vi "Dependency Add Source Path.vi"(7 "Source Path (relative)":string, 8 "error in (no error)":errorcluster, 10 "Dependency ref in":refnum<k20>, 11 "XML File ref in":refnum<k20>) -> (0 "error out":errorcluster, 2 "Dependency ref out":refnum<k20>, 3 "XML File ref out":refnum<k20>)   [LabVIEW 2020, in "LVLIBP CD XML Updater.lvlib" / "Project XML Editor.lvclass"]
uses:
  Project XML Editor.lvclass
  <vilib>/xml/Close Reference(Node).vi
  <resource>/objmgr/DOMUserDefRef.rc
  <vilib>/xml/NI_XML.lvlib
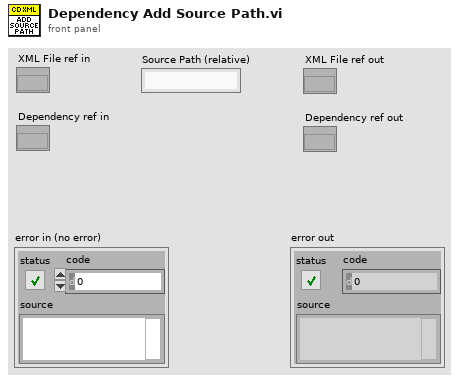
[diagram p1: front panel]
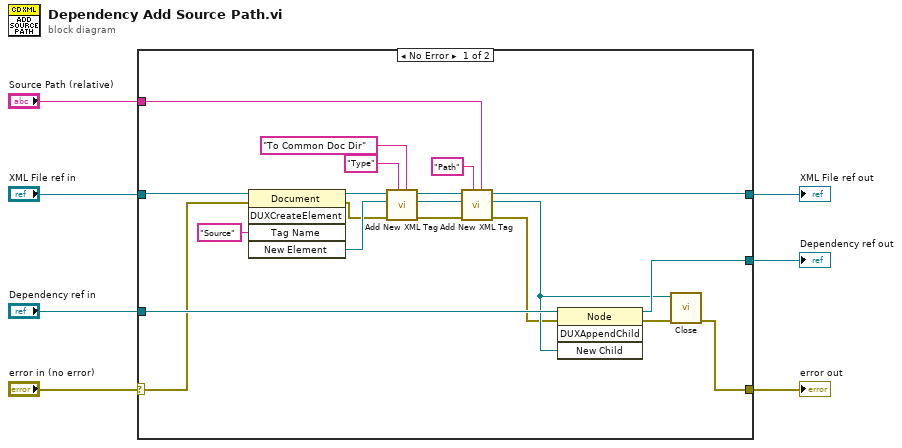
[diagram p0: block diagram]
diagram:
  n1 = case shown="No Error" "error in (no error)" {
    selector: "error in (no error)" -> [w13 w28]
    tunnel: "Source Path (relative)" -> [w19 _]
    tunnel: "XML File ref in" -> [w20 w29]
    tunnel: "Dependency ref in" -> [w18 w30]
    tunnel: [w17 w30] -> w4
    tunnel: [w16 w29] -> w3
    tunnel: [w9 w28] -> w2
    frame No Error {
      n2 = invoke class="Document" method="DUXCreateElement"(reference=w20, error in=w13, "Tag Name"="Source") -> (reference out=w22:refnum<k20>, error out=w12:errorcluster, "New Element"=w21:refnum<k20>)  [unwired: 2 in, 2 out]
      n3 = call "Add New XML Tag.vi"("Tag Data"="To Common Doc Dir", "Tag Name"="Type", "error in (no error)"=w12, "Owning Element"=w21, "XML File Ref in"=w22) -> ("error out"=w11:errorcluster, "dup Owning Element"=w26:refnum<k20>, "XML File Ref out"=w25:refnum<k20>)  [unwired: 4 in]
      n4 = call "Add New XML Tag.vi"("Tag Data"=w19, "Tag Name"="Path", "error in (no error)"=w11, "Owning Element"=w26, "XML File Ref in"=w25) -> ("error out"=w10:errorcluster, "dup Owning Element"=w15:refnum<k20>, "XML File Ref out"=w16:refnum<k20>)  [unwired: 4 in]
      n5 = invoke class="Node" method="DUXAppendChild"(reference=w18, error in=w10, "New Child"=w15) -> (reference out=w17:refnum<k20>, error out=w14:errorcluster)  [unwired: 1 in, 2 out]
      n6 = call-poly <vilib>:"Close.vi"("error in (no error)"=w14, "node"=w15) -> ("error out"=w9:errorcluster)  [unwired: 7 in]
    }
    frame Error {
    }
  }
  "Dependency ref out" <- w4
  "XML File ref out" <- w3
  "error out" <- w2
